vi "Power.vi"(8 "error in (no error)":errorcluster, 9 "Enable Drive":bool, 10 "Enable Axis":bool, 11 "SoftmotionAxis in":refnum<class "SoftmotionAxis.lvclass">) -> (0 "error out":errorcluster, 3 "SoftmotionAxis out":refnum<class "SoftmotionAxis.lvclass">)   [LabVIEW 2017, in "SoftmotionAxis.lvclass"]
uses:
  SoftmotionAxis.lvclass
  <resource>/objmgr/nimcai.rc
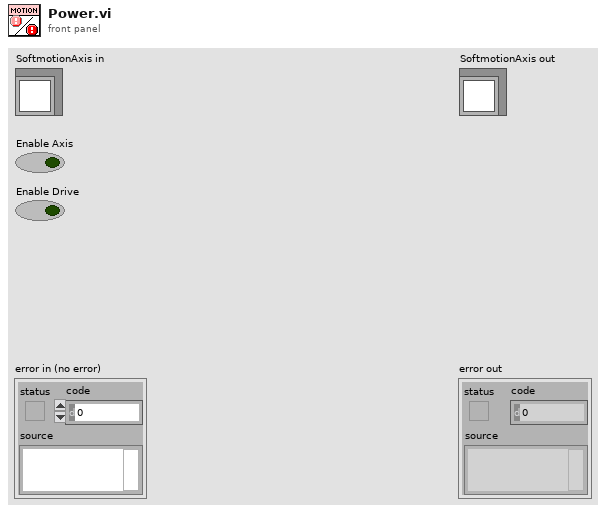
[diagram p1: front panel]
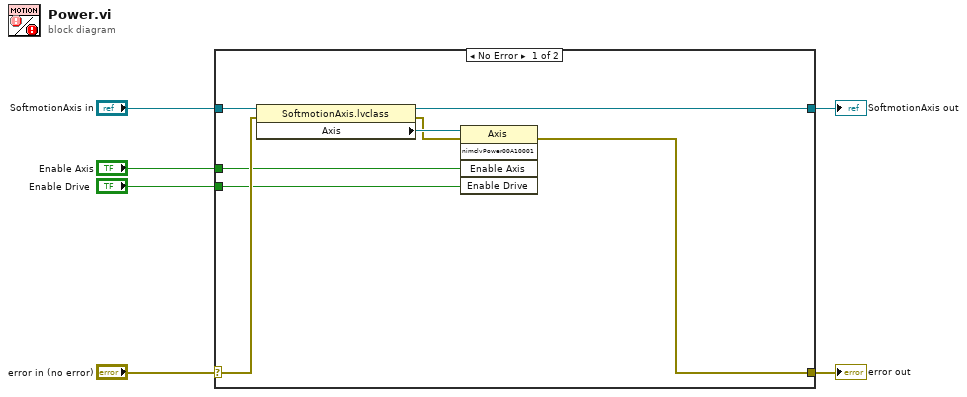
[diagram p0: block diagram]
diagram:
  n1 = case shown="No Error" "error in (no error)" {
    selector: "error in (no error)" -> [w10 w16]
    tunnel: [w9 w16] -> w5
    tunnel: [w13 w15] -> w3
    tunnel: "SoftmotionAxis in" -> [w14 w15]
    tunnel: "Enable Axis" -> [w8 _]
    tunnel: "Enable Drive" -> [w7 _]
    frame No Error {
      n2 = property class="SoftmotionAxis.lvclass"(reference=w14, error in=w10) -> (reference out=w13:refnum<class "SoftmotionAxis.lvclass">, error out=w11:errorcluster, "Axis"=w12:refnum<k21>)
      n3 = invoke class="Axis" method="nimclvPower00A10001"(reference=w12, error in=w11, "Enable Axis"=w8, "Enable Drive"=w7) -> (error out=w9:errorcluster)  [unwired: 1 in, 4 out]
    }
    frame Error {
    }
  }
  "error out" <- w5
  "SoftmotionAxis out" <- w3
